vi "Init.vi"(8 "error in (no error)":errorcluster, 11 "uService Template in":refnum<class "Kasli Server.lvclass">) -> (0 "error out":errorcluster, 3 "uService Template out":refnum<class "Kasli Server.lvclass">)   [LabVIEW 2020, in "Kasli Server.lvlib" / "Kasli Server.lvclass"]
uses:
  Kasli Server.lvclass
  Father of all uServices/Father of all uServices/Father of all uServices.lvclass
  Ancestor/Ancestor/Ancestor.lvclass
  C:/Users/marco/Documents/GitHub_Lab/TALOS/talos/Father of all uServices/Father of all uServices/Father of all uServices.lvclass
  C:/Users/marco/Documents/GitHub_Lab/TALOS/talos/Ancestor/Ancestor/Ancestor.lvclass
  C:/Users/marco/Documents/GitHub_Lab/TALOS/builds/Actor Framework PPL/Actor Framework.lvlibp/1abvi3w/vi.lib/ActorFramework/Actor/Actor.lvclass
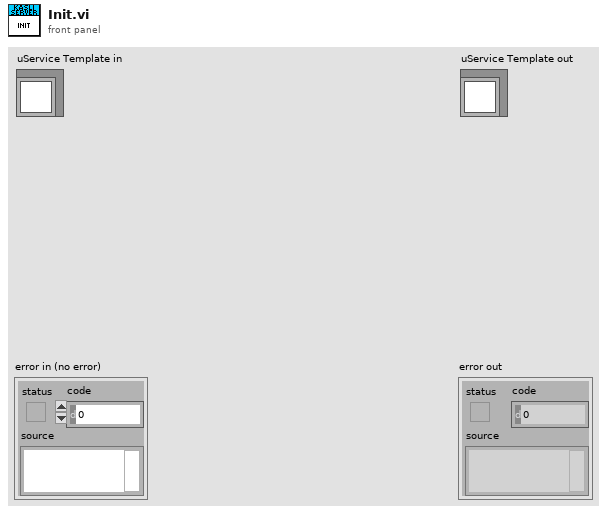
[diagram p1: front panel]
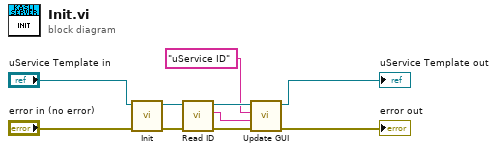
[diagram p0: block diagram]
diagram:
  n1 = call-parent "Init.vi"("error in (no error)"="error in (no error)", "uService Template in"="uService Template in") -> ("error out"=w7:errorcluster, "uService Template out"=w8:refnum<class "Kasli Server.lvclass">)  [unwired: 8 in]
  n2 = call "Read ID.vi"("error in (no error)"=w7, "Ancestor in"=w8) -> ("error out"=w6:errorcluster, "ID"=w3:string, "Ancestor out"=w5:refnum<class "Kasli Server.lvclass">)  [unwired: 7 in]
  n3 = call "Update GUI.vi"("error in (no error)"=w6, "Data"=w3, "GUI Item Name"="uService ID", "uService Template in"=w5) -> ("error out"=→"error out":errorcluster, "uService Template out"=→"uService Template out":refnum<class "Kasli Server.lvclass">)  [unwired: 6 in]
